vi "SaveToFile.vi"(6 "Overwrite":bool, 8 "Error In":errorcluster, 9 "File Path":path, 10 "Journal":refnum<class "Journal.lvclass">, 11 "Persistance":refnum<class "Persistence.lvclass">) -> (0 "Error Out":errorcluster)   [LabVIEW 2018, in "Persistence.lvclass"]
uses:
  Persistence.lvclass
  Journal/Journal.lvclass
  Journal/Journal.lvclass/Journal.ctl
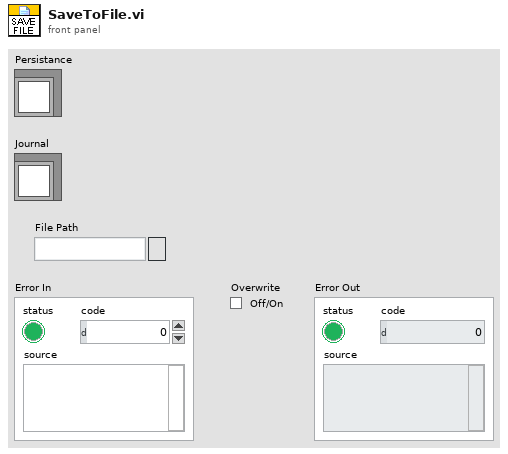
[diagram p1: front panel]
types:
  T1 = enum16{"open", "replace", "create", "open or create", "replace or create", "replace or create with confirmation"}
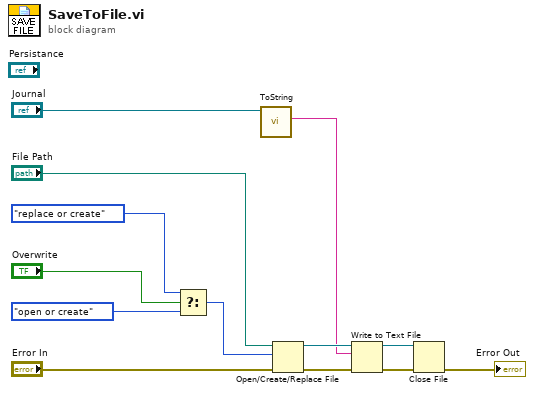
[diagram p0: block diagram]
diagram:
  n1 = Select(t=T1."replace or create" ("operation (0:open)"), s="Overwrite", f=T1."open or create" ("operation (0:open)")) -> (s? t:f=w10:T1)
  n2 = call "ToString.vi"("Journal In"="Journal") -> ("String"=w4:string)  [unwired: 9 in, 1 out]
  n3 = Open/Create/Replace File(file path (use dialog)="File Path", error in="Error In", operation (0:open)=w10) -> (refnum out=w8:refnum<file>, error out=w6:errorcluster)  [unwired: 3 in, 1 out]
  n4 = Write to Text File(file (use dialog)=w8, text=w4, error in=w6) -> (refnum out=w3:refnum<file>, error out=w2:errorcluster)  [unwired: 1 in, 1 out]
  n5 = Close File(refnum=w3, error in=w2) -> (error out=→"Error Out":errorcluster)  [unwired: 1 out]
